vi "Scan_1SDI_v00.vi"(8 "Scan (-1)":fxp<+,33,17> format="%.22g", 9 "Scan out (-1)":i16, 11 "Control Cavity":T1={"Lock"=FALSE, "Hold"=FALSE, "P Gain"=0, "P BS"=-5, "I Gain"=0, "I BS"=-10, "I2 G"=0, "I2 BS"=-26, "Scan Amp"=0, "Scan Off"=0, "Scan FS"=0, "SFS BS"=0, "I Max value"=10000, "I2 Max value"=10000, "Scope.Offset"=0, "Trigger Direction"=enum."either", "Scan-PII thresh"=0}) -> (0 "Scan":fxp<+,33,17> format="%.22g", 1 "Scan out":i16, 3 "Zero Crossing":bool)   [LabVIEW 2011]
doc: "Produces a variable saw tooth wave used for scanning the phase between two interfering beams. Based on a Look-Up-Table. Original design by Ben Sparkes."
uses:
  Strict Type Defs/PII individual.ctl
  <vilib>/rvi/Analysis/common/FxpNativeNode/niFpgaFxpNative.xnode
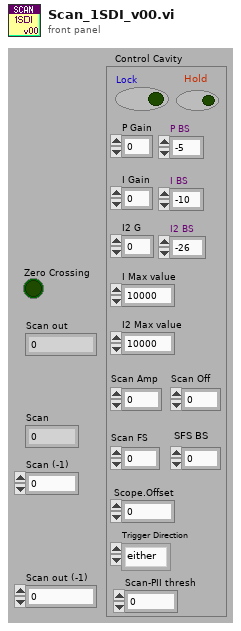
[diagram p1: front panel]
types:
  T1 = typedef "PII individual.ctl" = cluster{"Lock":bool, "Hold":bool, "P Gain":i32, "P BS":i16, "I Gain":i32, "I BS":i16, "I2 G":i32, "I2 BS":i16, "Scan Amp":i16, "Scan Off":i16, "Scan FS":u16, "SFS BS":i16, "I Max value":i32, "I2 Max value":i32, "Scope.Offset":i16, "Trigger Direction":enum8{"either", "minus-plus", "plus-minus"}, "Scan-PII thresh":i16}
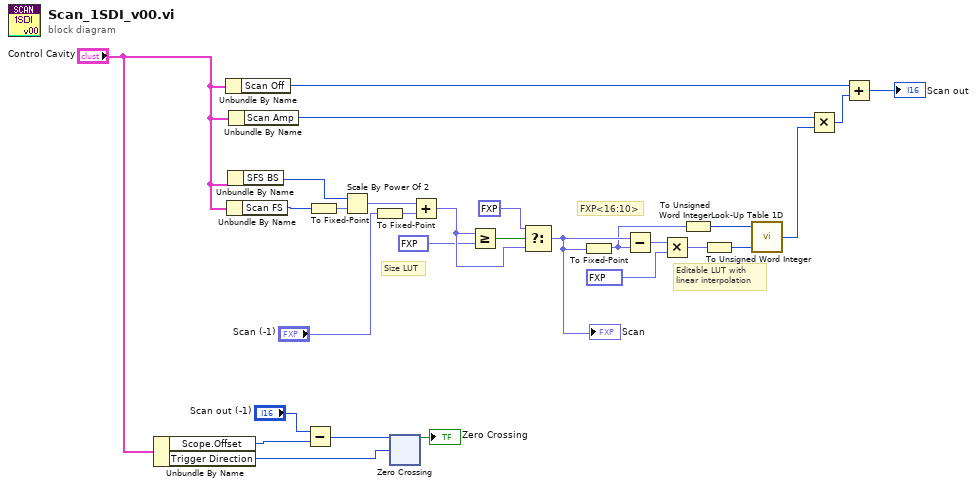
[diagram p0: block diagram]
diagram:
  # "FXP<16:10>"
  # "Size LUT"
  # "Editable LUT with \nlinear interpolation"
  n1 = Unbundle By Name("Control Cavity") -> ("Scope.Offset"=w23:i16, "Trigger Direction"=w21:enum8{"either", "minus-plus", "plus-minus"})
  n2 = Unbundle By Name("Control Cavity") -> ("Scan Off"=w26:i16)
  n3 = Unbundle By Name("Control Cavity") -> ("Scan FS"=w5:u16)
  n4 = Unbundle By Name("Control Cavity") -> ("SFS BS"=w4:i16)
  n5 = Unbundle By Name("Control Cavity") -> ("Scan Amp"=w28:i16)
  n6 = Subtract(x="Scan out (-1)", y=w23) -> (x-y=w22:i16)
  n7 = To Fixed-Point(number=w5) -> (fixed-point=w8:fxp<+,32,16>)  [unwired: 1 out]
  n8 = Scale By Power Of 2(n=w4, x=w8) -> (x*2^n=w7:fxp<+,32,16>)
  n9 = To Fixed-Point(number="Scan (-1)") -> (fixed-point=w9:fxp<+,32,16>)  [unwired: 1 out]
  n10 = xnode ("Zero Crossing")("direction"=w21, "input"=w22) -> ("crossing"=→"Zero Crossing":bool)  [unwired: 1 in]
  n11 = Add(x=w7, y=w9) -> (x+y=w18:fxp<+,33,17>)
  n12 = Greater Or Equal?(x=w18, y=fxp<+,17,17> 2000.0) -> (x >= y?=w11:bool)
  n13 = Select(t=fxp<+,33,17> 0.0, s=w11, f=w18) -> (s? t:f=w19:fxp<+,33,17>)
  "Scan" <- w19
  n14 = To Fixed-Point(number=w19) -> (fixed-point=w17:fxp<+,16,16>)  [unwired: 1 out]
  n15 = Subtract(x=w19, y=w17) -> (x-y=w12:fxp<+/-,34,18>)
  n16 = Multiply(x=w12, y=fxp<+/-,27,27> 65536.0) -> (x*y=w14:fxp<+/-,60,44>)
  n17 = To Unsigned Word Integer(number=w17) -> (unsigned 16bit integer=w16:u16)
  n18 = To Unsigned Word Integer(number=w14) -> (unsigned 16bit integer=w15:u16)
  n19 = call "Look-Up Table 1D"("address"=w16, "fractional index (x 2^16)"=w15) -> ("data out"=w2:i16)  [unwired: 7 out]
  n20 = Multiply(x=w28, y=w2) -> (x*y=w27:i16)
  n21 = Add(x=w26, y=w27) -> (x+y=→"Scan out":i16)
